vi "Read_many_files.vi"() -> ()   [LabVIEW 2010]
panel:
  out "Numeric":i32
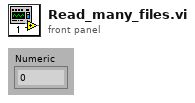
[diagram p1: front panel]
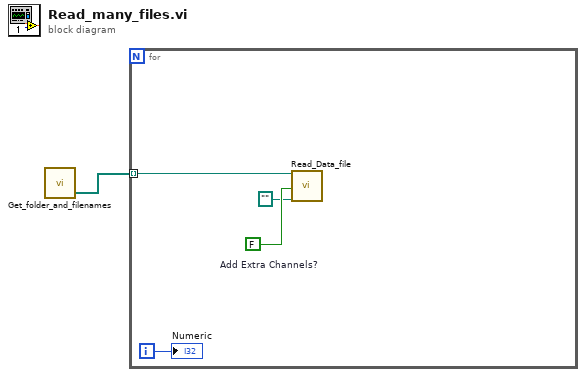
[diagram p0: block diagram]
diagram:
  n1 = call "Get_folder_and_filenames.vi"() -> ("Files"=w1:path[])  [unwired: 1 in, 1 out]
  n2 = for {
    tunnel: w1 -> [w3] mode=indexing
    i -> [w2]
    w5 = FALSE  # Add Extra Channels?
    n3 = call "Read_Data_file.vi"("Results file"=w3, "Add Extra Channels?"=w5, "Template File"=path "") -> ()  [unwired: 7 in, 10 out]
    "Numeric" <- w2
  }
